vi "Easy PID.vi"(4 "Back-Calculation Gain Kb (1)":dbl=1.0, 5 "Parallel Output":dbl, 6 "Anti-Windup Method (Clamping)":T2, 7 "Reset":bool, 8 "Process Variable":dbl, 9 "Setpoint":dbl, 10 "Output Range":T3, 11 "Gains":T1) -> (0 "Accumulator":dbl, 2 "Output":dbl)   [LabVIEW 2015, in "PID.lvlib"]
uses:
  PID.lvlib
  Output Range.ctl
  Anti-Windup Method.ctl
  Gains.ctl
  PID.ctl
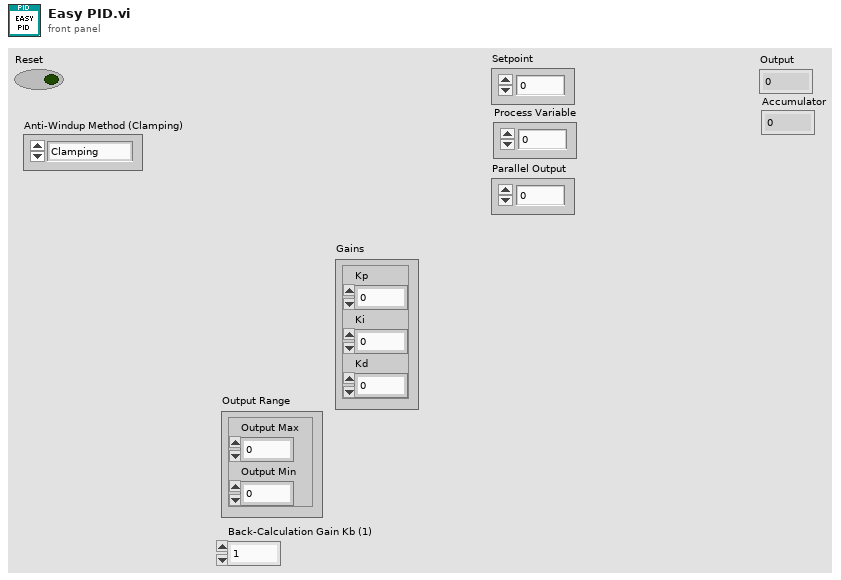
[diagram p1: front panel]
types:
  T1 = typedef "PID.lvlib/Gains.ctl" = cluster{"Kp":dbl, "Ki":dbl, "Kd":dbl}
  T2 = typedef "PID.lvlib/Anti-Windup Method.ctl" = enum16{"Clamping", "Back-Calculation", "None"}
  T3 = typedef "PID.lvlib/Output Range.ctl" = cluster{"Output Max":dbl, "Output Min":dbl}
  T4 = typedef "PID.lvlib/PID.ctl" = cluster{"Accumulator":dbl, "Kb":dbl, "Anti-Windup Method":T2, "Previous Error":dbl, "Gains":T1, "Output Range":T3}
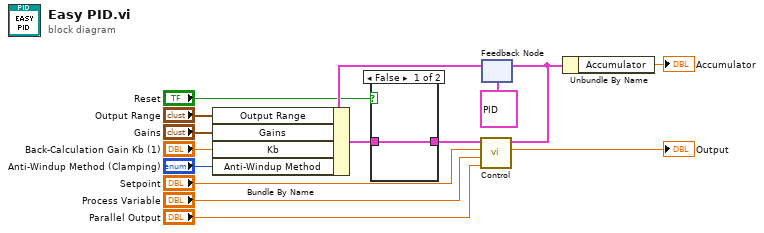
[diagram p0: block diagram]
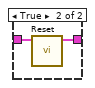
[diagram p2: hidden frame]
diagram:
  n1 = feedback #1(T4 {"Accumulator"=0.0, "Kb"=0.0, "Anti-Windup Method"=enum."Clamping", "Previous Error"=0.0, "Gains"={"Kp"=0.0, "Ki"=0.0, "Kd"=0.0}, "Output Range"={"Output Max"=0.0, "Output Min"=0.0}} ("PID out")) -> (w13:T4)
  n2 = Bundle By Name(cluster=w13, "Output Range"="Output Range", "Gains"="Gains", "Kb"="Back-Calculation Gain Kb (1)", "Anti-Windup Method"="Anti-Windup Method (Clamping)") -> (w5:T4)
  n3 = case shown="False" "Reset" {
    tunnel: [w16 w17] -> w6
    tunnel: w5 -> [w16 w18]
    frame False {
    }
    frame True {
      n4 = call "Reset.vi"("PID in"=w18) -> ("PID out"=w17:T4)  [unwired: 10 in]
    }
  }
  n5 = call "Control.vi"("Parallel Output"="Parallel Output", "Process Variable"="Process Variable", "Setpoint"="Setpoint", "PID in"=w6) -> ("Output"=→"Output":dbl, "PID out"=w2:T4)  [unwired: 6 in]
  n6 = feedback-in #1(w2) -> ()
  n7 = Unbundle By Name(w2) -> ("Accumulator"=→"Accumulator":dbl)
